vi "Lvdt data.vi"(11 "Lvdt":refnum<vi>) -> (0 "LVDT":bool, 1 "lvdt":dbl, 2 "lvdt":dbl format="%0.03f")   [LabVIEW 2020]
uses:
  Galobal variable_TI.vi
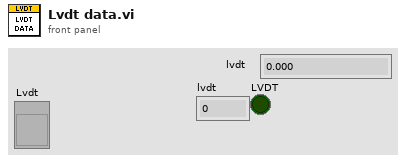
[diagram p1: front panel]
types:
  T1 = cluster{"MaxLoad ":dbl, "Min Load":dbl, "MaxDistance(mm)":dbl, "Min Distance(mm)":dbl, "Load Offset":dbl, "Model":string, "Difusser Code":string, "TFT Code ":string, "LVDT Offset":dbl}
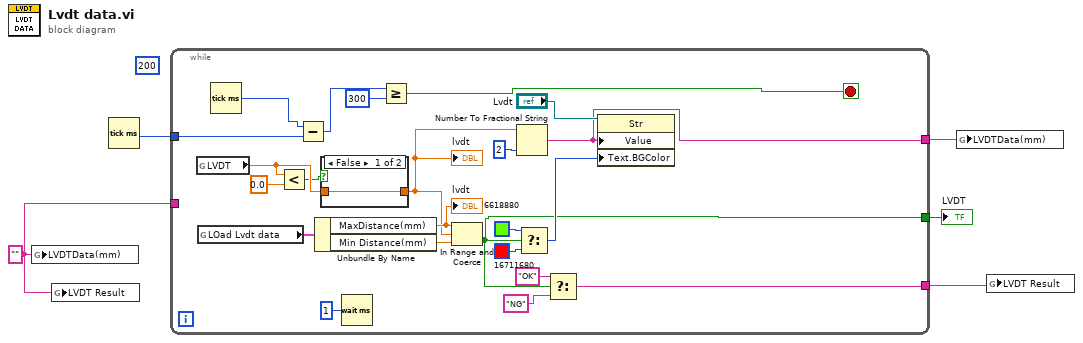
[diagram p0: block diagram]
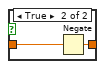
[diagram p2: hidden frame]
diagram:
  w1 = "" ("LVDTData(mm)")
  (unwired) 200
  n1 = global write "Galobal variable_TI.vi" "LVDTData(mm)"(w1) -> ()
  n2 = global write "Galobal variable_TI.vi" "LVDT Result"(w1) -> ()
  n3 = Tick Count (ms)() -> (millisecond timer value=w5:u32)
  n4 = while {
    tunnel: w5 -> [w19]
    tunnel: [w11] -> w4
    tunnel: [w14] -> w3
    tunnel: w1 -> [_]
    tunnel: [w10] -> w2
    stop <- w16 stop-if-true
    n5 = global read "Galobal variable_TI.vi" "LVDT"() -> (w8:dbl)
    n6 = global read "Galobal variable_TI.vi" "LOad Lvdt data"() -> (w23:T1)
    n7 = Tick Count (ms)() -> (millisecond timer value=w20:u32)
    n8 = Less?(x=w8, y=0.0) -> (x < y?=w7:bool)
    n9 = Subtract(x=w20, y=w19) -> (x-y=w18:u32)
    n10 = Unbundle By Name(w23) -> ("MaxDistance(mm)"=w22:dbl, "Min Distance(mm)"=w21:dbl)
    "lvdt" <- w22
    n11 = case shown="False" w7 {
      tunnel: w8 -> [w29 w31]
      tunnel: [w29 w30] -> w6
      frame False {
      }
      frame True {
        n12 = Negate(x=w31) -> (-x=w30:dbl)
      }
    }
    "lvdt" <- w6
    n13 = Wait (ms)(milliseconds to wait=u32 1) -> ()  [unwired: 1 out]
    n14 = Greater Or Equal?(x=w18, y=u32 300) -> (x >= y?=w16:bool)
    n15 = In Range and Coerce(upper limit=w22, x=w6, lower limit=w21) -> (In Range?=w11:bool)  [unwired: 1 out]
    n16 = Number To Fractional String(number=w6, precision (6)=i16 2) -> (F-format string=w14:string)  [unwired: 2 in]
    n17 = Select(t=u32 6618880, s=w11, f=u32 16711680) -> (s? t:f=w28:u32)
    n18 = Select(t="OK", s=w11, f="NG") -> (s? t:f=w10:string)
    n19 = property class="Str"(reference="Lvdt", "Value"=w14, "Text.BGColor"=w28) -> ()  [unwired: 1 in, 2 out]
  }
  "LVDT" <- w4
  n20 = global write "Galobal variable_TI.vi" "LVDTData(mm)"(w3) -> ()
  n21 = global write "Galobal variable_TI.vi" "LVDT Result"(w2) -> ()
